vi "Process Digital Configuration.vi"(7 "PMU Name":string, 11 "Digital Configuration In":T1) -> (2 "Digital Channel Names":string[](array[string]), 3 "Digital Configuration Out":T2(array[cluster]))   [LabVIEW 2013, in "PMU Recorder Light.lvlib" / "Phasor Data Concentrator.lvclass"]
uses:
  Phasor Data Concentrator.lvclass
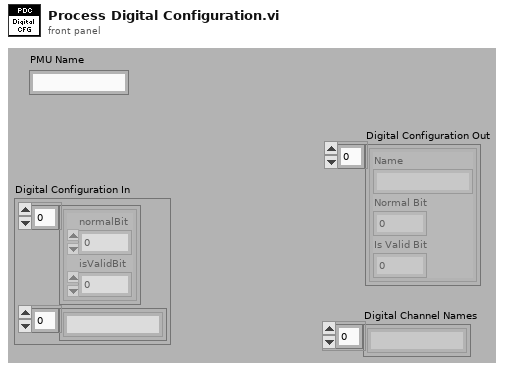
[diagram p1: front panel]
types:
  T1 = cluster{cluster{"normalBit":u8, "isValidBit":u8}[], string[]}
  T2 = cluster{"Name":string, "Normal Bit":u8, "Is Valid Bit":u8}[]
  T3 = cluster{"Name":string, "Normal Bit":u8, "Is Valid Bit":u8}
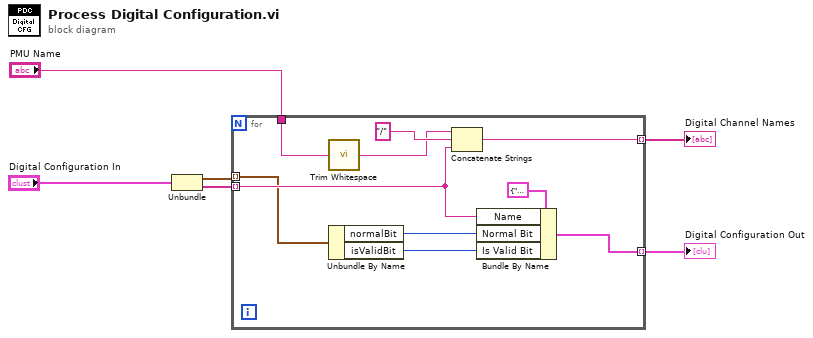
[diagram p0: block diagram]
diagram:
  n1 = Unbundle("Digital Configuration In") -> (w3:cluster{"normalBit":u8, "isValidBit":u8}[], w4:string[])
  n2 = for {
    tunnel: [w15] -> w6 mode=indexing
    tunnel: "PMU Name" -> [w13]
    tunnel: w4 -> [w12] mode=indexing
    tunnel: w3 -> [w11] mode=indexing
    tunnel: [w9] -> w2 mode=indexing
    n3 = call <vilib>:"Trim Whitespace.vi"("string"=w13) -> ("trimmed string"=w14:string)  [unwired: 1 in]
    n4 = Unbundle By Name(w11) -> ("normalBit"=w7:u8, "isValidBit"=w10:u8)
    n5 = Concatenate Strings(w14, "/" ("string"), w12) -> (w15:string)
    n6 = Bundle By Name(cluster=T3 {"Name"="", "Normal Bit"=0, "Is Valid Bit"=0} ("Digital Configuration"), "Name"=w12, "Normal Bit"=w7, "Is Valid Bit"=w10) -> (w9:T3)
  }
  "Digital Channel Names" <- w6
  "Digital Configuration Out" <- w2
